vi "Clear Illegal Characters.vi"(11 "String in":string) -> (3 "Safe String out":string)   [LabVIEW 2023, in "Report.lvlib" / "Report.lvclass"]
uses:
  Report.lvclass
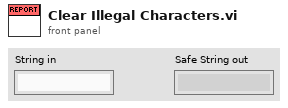
[diagram p1: front panel]
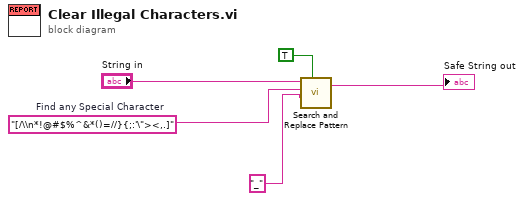
[diagram p0: block diagram]
diagram:
  w5 = "[/\\n*!@#$%^&*()=//}{;:'\"><,.]"  # Find any Special Character
  n1 = call <vilib>:"Search and Replace Pattern.vi"("string"="String in", "regular expression (\"\")"=w5, "replace string (\"\")"="_" ("replace string (\"\")"), "replace all? (F)"=TRUE) -> ("result string"=→"Safe String out":string)  [unwired: 1 in, 1 out]
